vi "34970 Reset Instrument.vi"(0 "VISA resource name":refnum<visa-resource-name>, 11 "error in (no error)":errorcluster) -> (4 "VISA resource name out":refnum<visa-resource-name>, 15 "error out":errorcluster)   [LabVIEW 2020]
doc: "Issues only a configuration Reset command(see p 160 34970 user manual)\nW. Gilbert, University of Minnesota Physics, 8/6/2004\nwgilbert@physics.umn.edu"
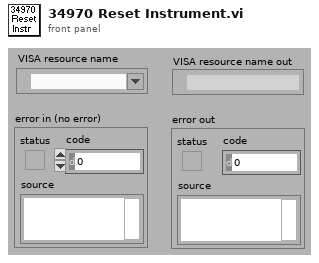
[diagram p1: front panel]
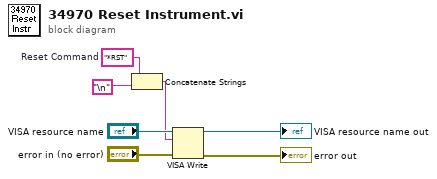
[diagram p0: block diagram]
diagram:
  w2 = "*RST"  # Reset Command
  n1 = Concatenate Strings(w2, "\n") -> (w3:string)
  n2 = VISA Write(VISA resource name="VISA resource name", write buffer=w3, error in (no error)="error in (no error)") -> (VISA resource name out=→"VISA resource name out":refnum<visa-resource-name>, error out=→"error out":errorcluster)  [unwired: 1 out]
